vi "LMS on SW Map 3.vi"(8 "SW Map In":i32[][](array[numeric]), 11 "LMS Vector":dbl[](array[numeric])) -> (3 "SW Map Out":i32[][](array[numeric]))   [LabVIEW 2014]
panel:
  out "LMS Vector Check":dbl[](array[numeric])
  out "Test SW Map Out of y":dbl[](array[numeric])
  out "Test SW Map Out of x":dbl[](array[numeric])
  # "LMS on SW Map 3"
  # "Inputs:"
  # "Outputs:"
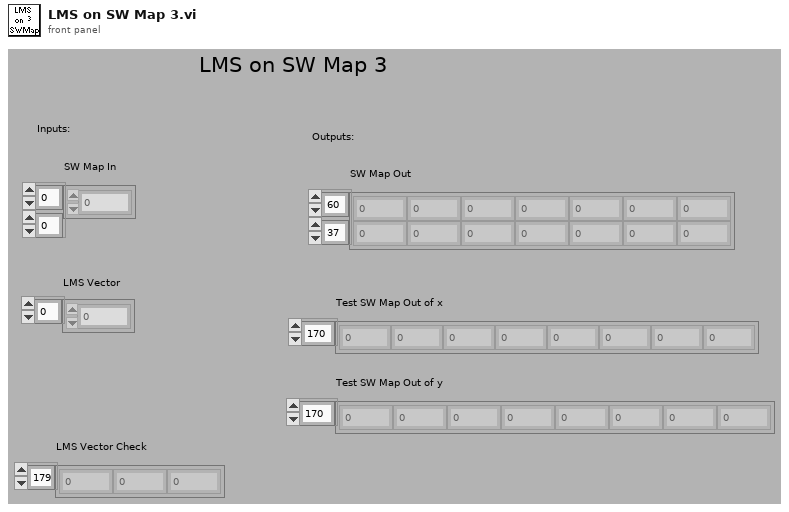
[diagram p1: front panel]
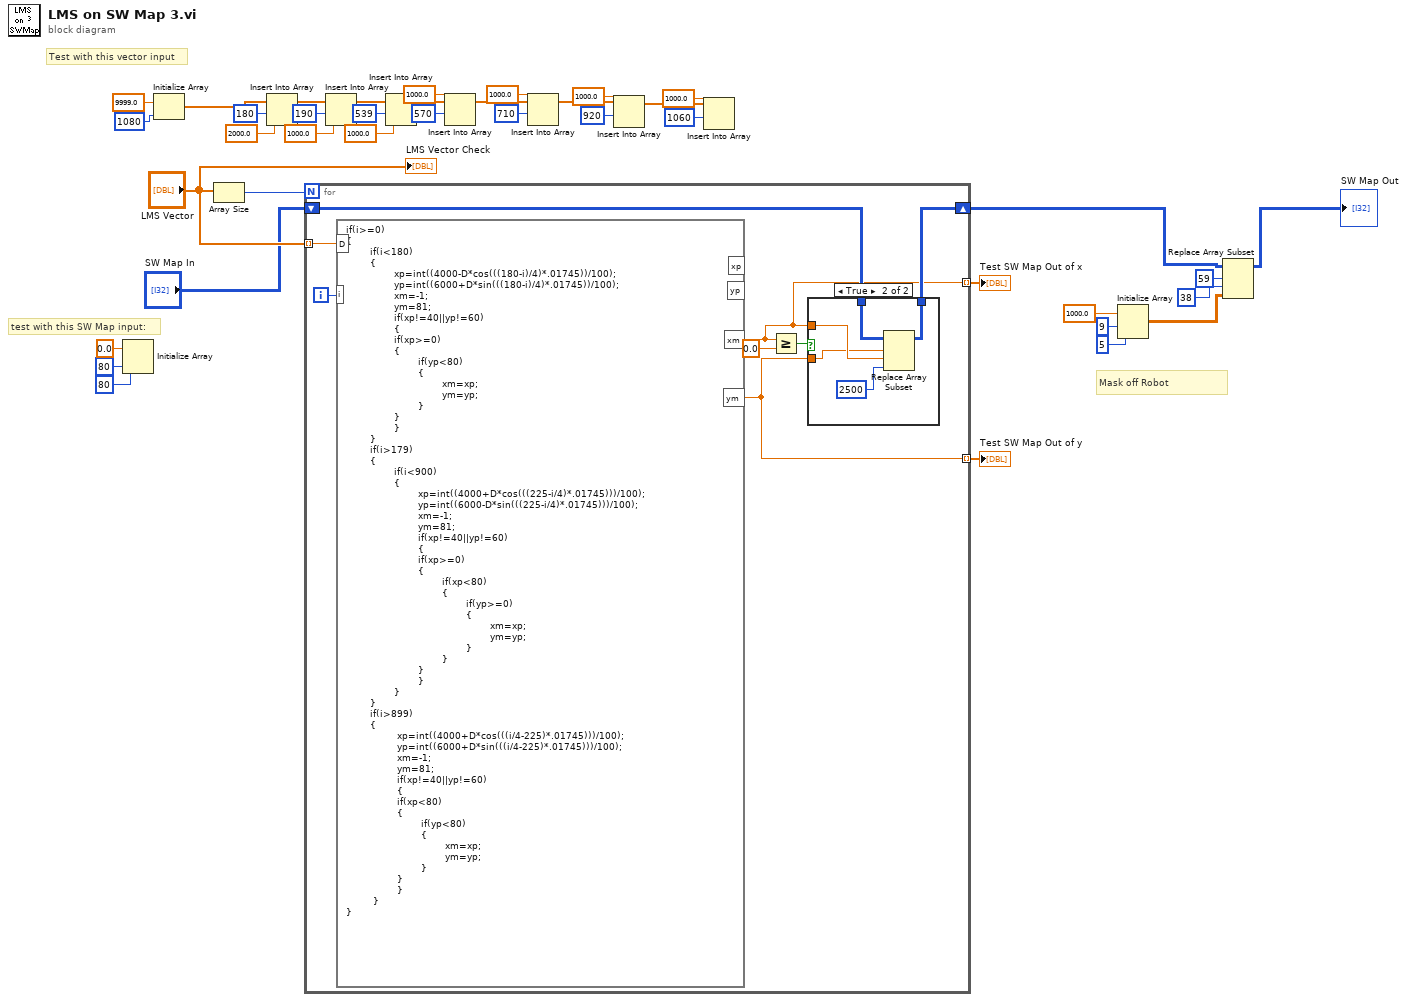
[diagram p0: block diagram]
diagram:
  # "Mask off Robot"
  # "test with this SW Map input:"
  # "Test with this vector input"
  n1 = Initialize Array(0.0 ("element"), 80 ("dimension size"), 80 ("dimension size")) -> ()  [unwired: 1 out]
  n2 = Initialize Array(9999.0 ("element"), 1080 ("dimension size")) -> (w38:dbl[])
  n3 = Array Size(array="LMS Vector") -> (size(s)=w36:i32)
  n4 = Insert Into Array(array=w38, index=180 ("index (row)"), new element=2000.0 ("new element/subarray")) -> (w11:dbl[])
  n5 = for {
    N: w36 -> [_]
    tunnel: "LMS Vector" -> [w47] mode=indexing
    shift-right: [w42] -> w5
    shift-left: "SW Map In" -> [w45]
    tunnel: [w41] -> w16 mode=indexing
    tunnel: [w40] -> w15 mode=indexing
    i -> [w46]
    n6 = formula code="if(i>=0) \n{\n        if(i<180)\n        {\n                xp=int((4000-D*cos(((180-i)/4)*.01745))/100);\n                yp=int((6000+D*sin(((180-i)/4)*.01745))/100);\n                xm=-1;\n                ym=81;\n                if(xp!=40||yp!=60)\n                {\n                if(xp>=0)\n                {\n                        if(yp<80)\n                        {\n                                xm=xp;\n                                ym=yp;\n                        }\n                }\n                }\n        }\n        if(i>179)\n        {\n                if(i<900)\n                {\n                        xp=int((4000+D*cos(((225-i/4)*.01745)))/100);\n                        yp=int((6000-D*sin(((225-i/4)*.01745)))/100);\n                        xm=-1;\n                        ym=81;\n                        if(xp!=40||yp!=60)\n                        {\n                        if(xp>=0)\n                        {\n                                if(xp<80)\n                                {\n                                        if(yp>=0)\n                                        {\n                                                xm=xp;\n                                                ym=yp;\n                                        }\n                                }\n                        }\n                        }\n                }\n        }\n        if(i>899)\n        {\n                 xp=int((4000+D*cos(((i/4-225)*.01745)))/100);\n                 yp=int((6000+D*sin(((i/4-225)*.01745)))/100);\n                 xm=-1;\n                 ym=81;\n                 if(xp!=40||yp!=60)\n                 {\n                 if(xp<80)\n                 {\n                         if(yp<80)\n                         {\n                                 xm=xp;\n                                 ym=yp;\n                         }\n                 }\n                 }\n         }\n}"("D"=w47, "i"=w46) -> ("xm"=w40:dbl, "ym"=w41:dbl)  [unwired: 2 out]
    n7 = Greater Or Equal?(x=w40, y=0.0) -> (x >= y?=w43:bool)
    n8 = case shown="True" w43 {
      tunnel: w45 -> [w48 w53]
      tunnel: [w48 w52] -> w42
      tunnel: w41 -> [_ w49]
      tunnel: w40 -> [_ w50]
      frame False {
      }
      frame True {
        n9 = Replace Array Subset(array=w53, new element=2500, index (row)=w49, index (col)=w50) -> (w52:i32[][])
      }
    }
  }
  "Test SW Map Out of x" <- w15
  "Test SW Map Out of y" <- w16
  n10 = Insert Into Array(array=w11, index=190, new element=1000.0 ("new element/subarray")) -> (w31:dbl[])
  n11 = Insert Into Array(array=w31, index=539, new element=1000.0 ("new element/subarray")) -> (w28:dbl[])
  n12 = Insert Into Array(array=w28, index=570, new element=1000.0 ("new element/subarray")) -> (w25:dbl[])
  n13 = Insert Into Array(array=w25, index=710, new element=1000.0 ("new element/subarray")) -> (w22:dbl[])
  n14 = Insert Into Array(array=w22, index=920, new element=1000.0 ("new element/subarray")) -> (w19:dbl[])
  n15 = Insert Into Array(array=w19, index=1060, new element=1000.0 ("new element/subarray")) -> ()  [unwired: 1 out]
  n16 = Initialize Array(1000.0 ("element"), 9 ("dimension size"), 5 ("dimension size")) -> (w3:dbl[][])
  n17 = Replace Array Subset(array=w5, new element=w3, index (row)=59, index (col)=38 ("disabled index (col)")) -> (→"SW Map Out":i32[][])
  "LMS Vector Check" <- "LMS Vector"
